vi "GetBarcodeResult.vi"(11 "掃碼R結果":string) -> (1 "state":i16, 3 "light":i16)   [LabVIEW 2019]
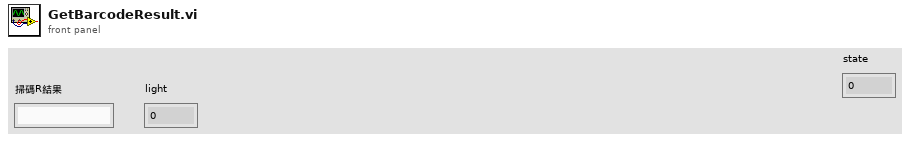
[diagram p1: front panel]
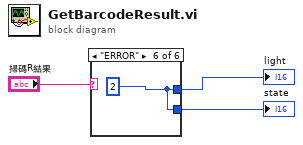
[diagram p0: block diagram]
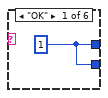
[diagram p2: hidden frame]
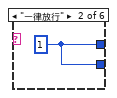
[diagram p3: hidden frame]
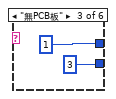
[diagram p4: hidden frame]
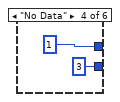
[diagram p5: hidden frame]
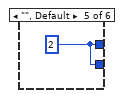
[diagram p6: hidden frame]
diagram:
  n1 = case shown="\"ERROR\"" "掃碼R結果" {
    tunnel: [w4 w5 i16 1 i16 1 w10 w11] -> w3
    tunnel: [w4 w5 i16 3 i16 3 w10 w11] -> w1
    frame "OK" {
      w4 = i16 1
    }
    frame "一律放行" {
      w5 = i16 1
    }
    frame "無PCB板" {
    }
    frame "No Data" {
    }
    frame "", Default {
      w10 = i16 2
    }
    frame "ERROR" {
      w11 = i16 2
    }
  }
  "light" <- w3
  "state" <- w1
